vi "local variables.vi"() -> ()   [LabVIEW 2024]
panel:
  out "Numeric":dbl
  in  "Knob":dbl(knob) scale=0.0..10.0
  in  "stop 2":bool
  in  "stop":bool
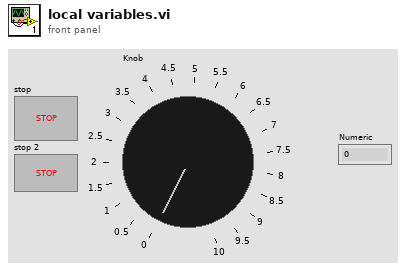
[diagram p1: front panel]
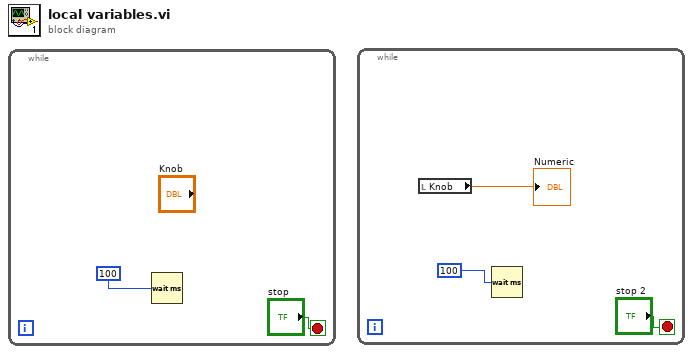
[diagram p0: block diagram]
diagram:
  n1 = while {
    stop <- "stop" stop-if-true
    n2 = Wait (ms)(milliseconds to wait=u32 100) -> ()  [unwired: 1 out]
  }
  n3 = while {
    stop <- "stop 2" stop-if-true
    n4 = local read "Knob"() -> (→"Numeric":dbl)
    n5 = Wait (ms)(milliseconds to wait=u32 100) -> ()  [unwired: 1 out]
  }
